vi "Signal Average_x.vi"(11 "Filtered Correction":dbl=0.1 format="%#_13g") -> (3 "Average Signal":dbl)   [LabVIEW 2019]
panel:
  in  "iterations":i32=100
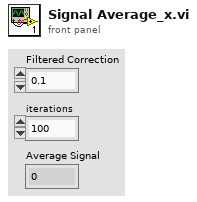
[diagram p1: front panel]
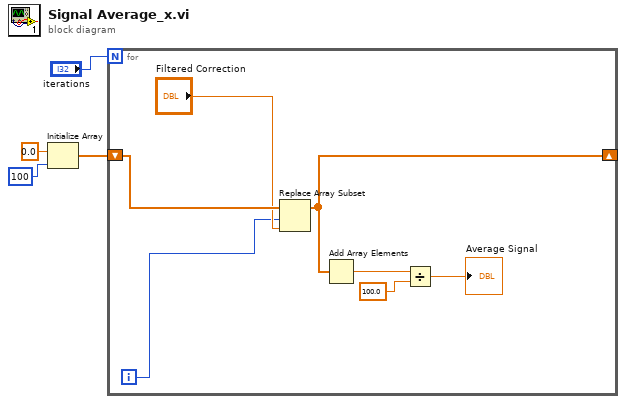
[diagram p0: block diagram]
diagram:
  n1 = Initialize Array(0.0 ("element"), 100 ("dimension size")) -> (w1:dbl[])
  n2 = for {
    N: "iterations" -> [_]
    shift-right: [w9] -> _
    shift-left: w1 -> [w11]
    i -> [w5]
    n3 = Replace Array Subset(array=w11, new element="Filtered Correction", index=w5) -> (w9:dbl[])
    n4 = Add Array Elements(numeric array=w9) -> (sum=w8:dbl)
    n5 = Divide(x=w8, y=100.0) -> (x/y=→"Average Signal":dbl)
  }
